vi "Transition Measurements 1 chan (obs).vi"(6 "percent level settings":T2={"method"=enum."auto select", "histogram size"=256, "histogram method"=enum."mode", "reserved"=1.0} {"reserved" format="%0.2f"}, 7 "edge number (1)":i32=1 min=1, 8 "error in (no error)":errorcluster, 9 "reference levels":T3={"high ref level"=90.0, "mid ref level"=50.0, "low ref level"=10.0, "ref units"=1} {"ref units" items=["absolute", "percent"]; "high ref level" format="%0.2f"; "low ref level" format="%0.2f"; "mid ref level" format="%0.2f"}, 10 "polarity (rising)":u16(ring)=1 items=["falling", "rising"], 11 "signal in":waveform(dbl)={"t0"=timestamp(0 s since 1904-01-01), "dt"=0.0, "Y"=[]}) -> (0 "error out":errorcluster, 1 "overshoot (%)":dbl format="%.2g", 2 "preshoot (%)":dbl format="%.2g", 3 "duration":dbl format="%.2g", 4 "measurement info":T1 {"ref levels"."ref units" items=["absolute", "relative"]; "ref levels"."high ref level" format="%.2p"; "ref levels"."low ref level" format="%.2p"; "ref levels"."mid ref level" format="%.2p"; "end time" format="%.2p"; "start time" format="%.2p"}, 5 "slew rate":dbl format="%.2g")   [LabVIEW 2020, in "NI_MAPro.lvlib"]
uses:
  NI_MAPro.lvlib
panel:
  # "This VI is obsolete !!!\nYou should replace this VI in your diagram with the Transition Measurements VI.  \n\nNOTE: If you have wired to the output of this obsolete VI, \n           please be aware that the new Transition Measurements VI:\n           1. Use two new clusters, pre-transition and under-transtion, to replace preshoot(%) and overshoot(%).\n           2. Change the output name slew rate to slope.\n           3. Change the output name duration to transition duration."
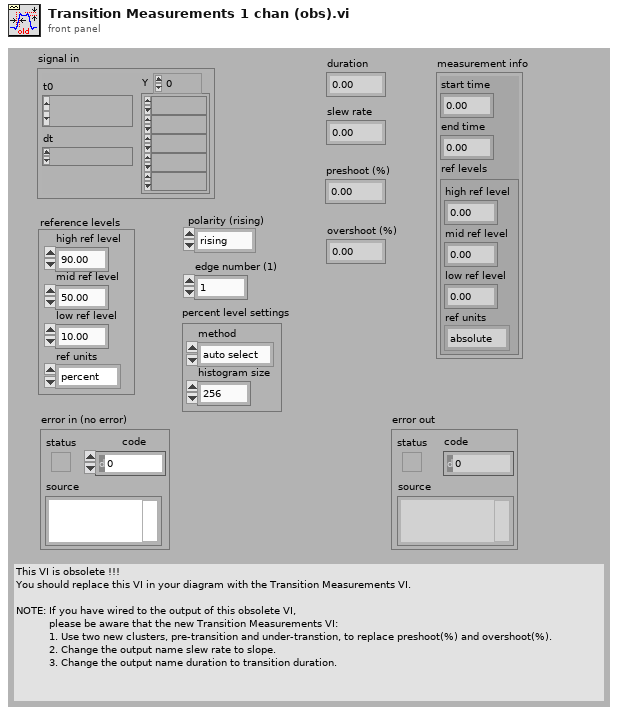
[diagram p1: front panel]
types:
  T1 = cluster{"start time":dbl, "end time":dbl, "ref levels":cluster{"high ref level":dbl, "mid ref level":dbl, "low ref level":dbl, "ref units":u16}}
  T2 = cluster{"method":enum32{"histogram", "peak", "auto select"}, "histogram size":i32, "histogram method":enum16{"mode"}, "reserved":dbl}
  T3 = cluster{"high ref level":dbl, "mid ref level":dbl, "low ref level":dbl, "ref units":u16}
  T4 = cluster{"undershoot (%)":dbl, "overshoot (%)":dbl}
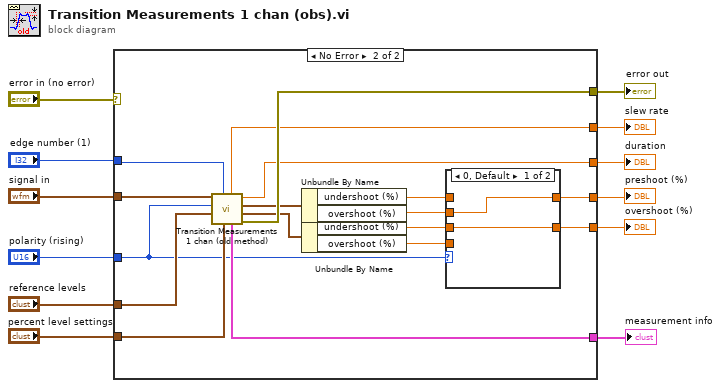
[diagram p0: block diagram]
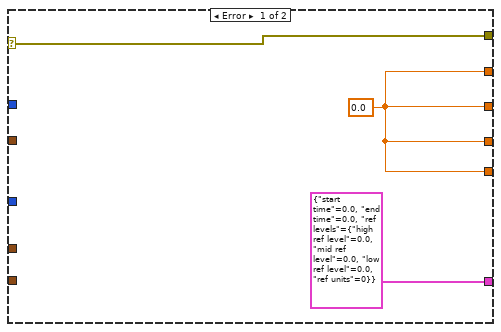
[diagram p2: hidden frame]
diagram:
  n1 = case shown="No Error" "error in (no error)" {
    selector: "error in (no error)" -> [w15 _]
    tunnel: "polarity (rising)" -> [_ w18]
    tunnel: "reference levels" -> [_ w31]
    tunnel: "percent level settings" -> [_ w25]
    tunnel: "edge number (1)" -> [_ w29]
    tunnel: "signal in" -> [_ w32]
    tunnel: [T1 {"start time"=0.0, "end time"=0.0, "ref levels"={"high ref level"=0.0, "mid ref level"=0.0, "low ref level"=0.0, "ref units"=0}} ("measurement info") w26] -> w1
    tunnel: [w15 w30] -> w6
    tunnel: [w13 w24] -> w5
    tunnel: [w13 w23] -> w4
    tunnel: [w13 w28] -> w3
    tunnel: [w13 w27] -> w2
    frame Error {
      w13 = 0.0 ("result")
    }
    frame No Error {
      n2 = call "Transition Measurements 1 chan (old method).vi"("percent level settings"=w25, "edge number (1)"=w29, "reference levels"=w31, "polarity (rising)"=w18, "signal in"=w32) -> ("error out"=w30:errorcluster, "post-transition"=w19:T4, "pre-transition"=w22:T4, "transition duration"=w23:dbl, "measurement info"=w26:T1, "slope"=w24:dbl)  [unwired: 1 in]
      n3 = Unbundle By Name(w22) -> ("undershoot (%)"=w21:dbl, "overshoot (%)"=w20:dbl)
      n4 = Unbundle By Name(w19) -> ("undershoot (%)"=w16:dbl, "overshoot (%)"=w17:dbl)
      n5 = case shown="0, Default" w18 {
        tunnel: w21 -> [_ w36]
        tunnel: w20 -> [w34 _]
        tunnel: w16 -> [w33 _]
        tunnel: w17 -> [_ w35]
        tunnel: [w34 w36] -> w28
        tunnel: [w33 w35] -> w27
        frame 0, Default {
        }
        frame 1 {
        }
      }
    }
  }
  "slew rate" <- w5
  "duration" <- w4
  "measurement info" <- w1
  "error out" <- w6
  "preshoot (%)" <- w3
  "overshoot (%)" <- w2
